vi "Contract Listbox.vi"(8 "error in (no error)":errorcluster, 11 "[V] Login in":refnum<class "[V] Login.lvclass">) -> (0 "error out":errorcluster, 3 "[V] Login out":refnum<class "[V] Login.lvclass">)   [LabVIEW 2020, in "[V] Login.lvlib" / "[V] Login.lvclass"]
uses:
  [V] Login.lvclass
  [V] Login.lvclass/[V] Login.ctl
  <vilib>/Analysis/1siggen.llb/Ramp Pattern by Samples.vi
  <vilib>/Analysis/NI_AALBase.lvlib
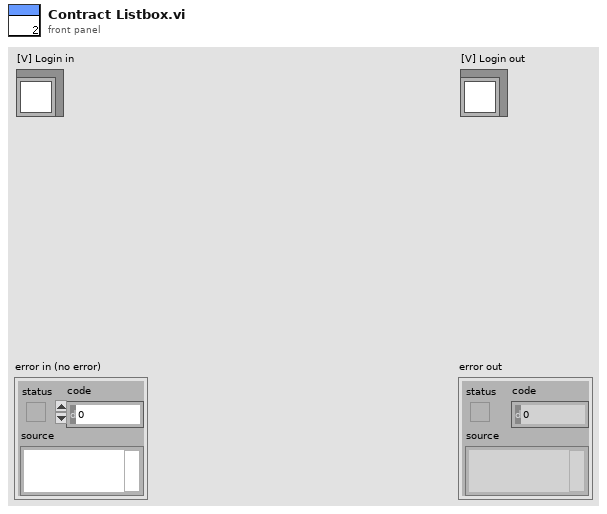
[diagram p1: front panel]
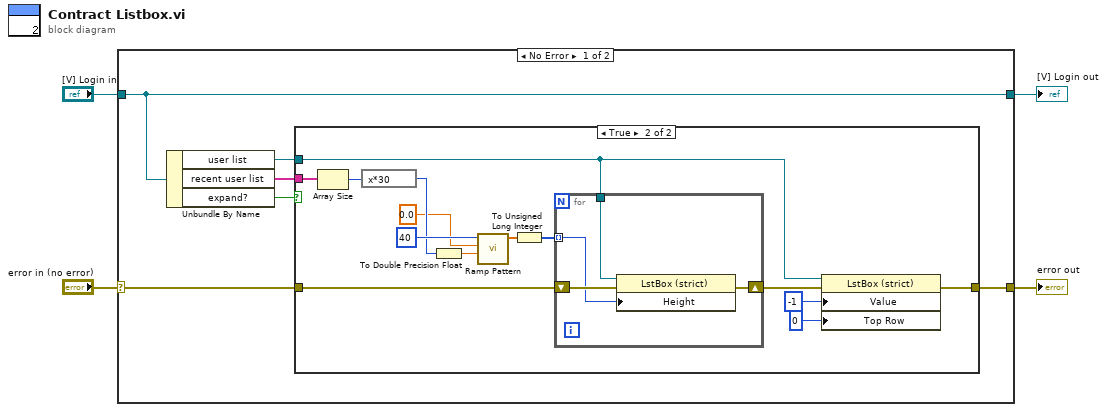
[diagram p0: block diagram]
diagram:
  n1 = case shown="No Error" "error in (no error)" {
    selector: "error in (no error)" -> [w10 w31]
    tunnel: [w8 w31] -> w3
    tunnel: [w9 w30] -> w1
    tunnel: "[V] Login in" -> [w9 w30]
    frame No Error {
      n2 = Unbundle By Name(w9) -> ("user list"=w7:refnum<vi>, "recent user list"=w6:string[], "expand?"=w5:bool)
      n3 = case shown="True" w5 {
        tunnel: w10 -> [w11 w24]
        tunnel: [w11 w20] -> w8
        tunnel: w7 -> [_ w19]
        tunnel: w6 -> [_ w16]
        frame False {
        }
        frame True {
          n4 = Array Size(array=w16) -> (size(s)=w15:i32)
          n5 = expression code="x*30"(w15) -> (w14:i32)
          n6 = To Double Precision Float(number=w14) -> (double precision float=w13:dbl)
          n7 = call-poly <vilib>:"Ramp Pattern.vi"("start"=w13, "end"=0.0 ("start"), "samples"=40) -> ("Ramp Pattern"=w23:dbl[])  [unwired: 7 in, 1 out]
          n8 = To Unsigned Long Integer(number=w23) -> (unsigned 32bit integer=w22:u32[])
          n9 = for {
            tunnel: w19 -> [w26]
            shift-right: [w28] -> w21
            shift-left: w24 -> [w29]
            tunnel: w22 -> [w27] mode=indexing
            n10 = property class="LstBox (strict)"(reference=w26, error in=w29, "Height"=w27) -> (error out=w28:errorcluster)  [unwired: 1 out]
          }
          n11 = property class="LstBox (strict)"(reference=w19, error in=w21, "Value"=-1, "Top Row"=0) -> (error out=w20:errorcluster)  [unwired: 1 out]
        }
      }
    }
    frame Error {
    }
  }
  "error out" <- w3
  "[V] Login out" <- w1
